vi "CalcArea.vi"(8 "Error In":errorcluster, 11 "Circle in":refnum<class "Circle.lvclass">) -> (0 "Error Out":errorcluster, 2 "Area":dbl, 3 "Circle out":refnum<class "Circle.lvclass">)   [LabVIEW 2021, in "Circle.lvclass"]
doc: "Calc a area of circle object."
uses:
  Circle.lvclass
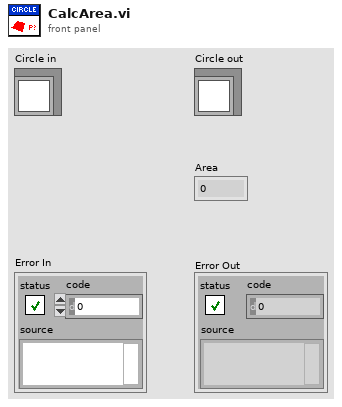
[diagram p1: front panel]
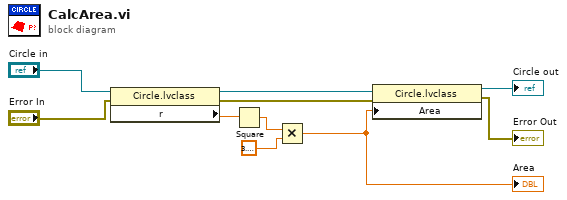
[diagram p0: block diagram]
diagram:
  n1 = property class="Circle.lvclass"(reference="Circle in", error in="Error In") -> (reference out=w5:refnum<class "Circle.lvclass">, error out=w4:errorcluster, "r"=w8:dbl)
  n2 = Square(x=w8) -> (x^2=w7:dbl)
  n3 = Multiply(x=w7, y=3.141592653589793) -> (x*y=w3:dbl)
  "Area" <- w3
  n4 = property class="Circle.lvclass"(reference=w5, error in=w4, "Area"=w3) -> (reference out=→"Circle out":refnum<class "Circle.lvclass">, error out=→"Error Out":errorcluster)
